vi "QTrkGetSingleResult.vi"(5 "QTrk Instance":T4={"QTrk Pointer"=0, "QTrk Settings"={"Image width"=150, "Image height"=150, "Number of threads (CPU based)"=-1, "Max Queue Size"=128, "XCOR Profile Length"=32, "XCOR Profile Width"=2, "XCOR Iterations"=5, "ZLUT MinRadius"=50.0, "ZLUT MaxRadius"=64.0, "ZLUT AngularSteps"=0, "QI Iterations"=64, "QI RadialSteps"=64, "QI AngularSteps Per Quadrant"=2, "QI MinRadius"=50.0, "QI MaxRadius"=50.0, "CUDA Device# (if using cuda)"=0, "COM Background correction factor"=2.0, "ZLUT RadialSteps"=32, "Gaussian 2D Fit Iterations"=8}}) -> (0 "HasResult":bool, 1 "result":T1, 2 "QTrk Instance":T4={"QTrk Pointer"=0, "QTrk Settings"={"Image width"=150, "Image height"=150, "Number of threads (CPU based)"=-1, "Max Queue Size"=128, "XCOR Profile Length"=32, "XCOR Profile Width"=2, "XCOR Iterations"=5, "ZLUT MinRadius"=50.0, "ZLUT MaxRadius"=64.0, "ZLUT AngularSteps"=0, "QI Iterations"=64, "QI RadialSteps"=64, "QI AngularSteps Per Quadrant"=2, "QI MinRadius"=50.0, "QI MaxRadius"=50.0, "CUDA Device# (if using cuda)"=0, "COM Background correction factor"=2.0, "ZLUT RadialSteps"=32, "Gaussian 2D Fit Iterations"=8}})   [LabVIEW 2011]
uses:
  QTrkInstance.ctl
  QTrkSettings.ctl
  QTrkLocalizationResult.ctl
  QTrkLocalizationJob.ctl
  XYZf.ctl
  QTrkDLL.vi
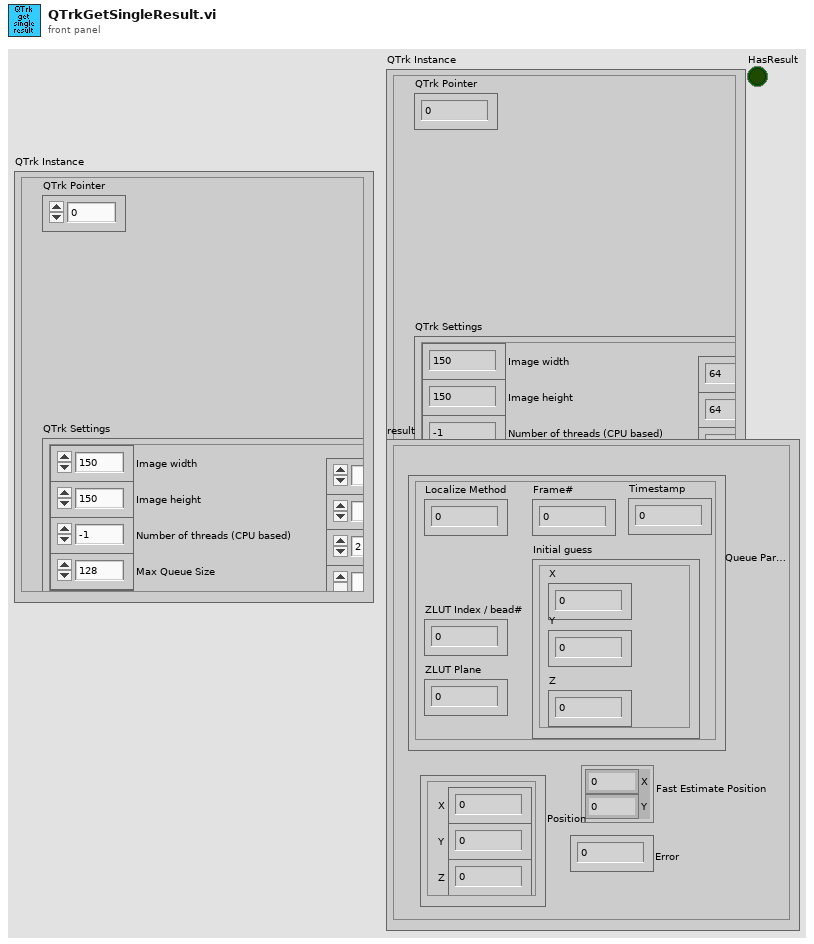
[diagram p1: front panel]
types:
  T1 = typedef "QTrkLocalizationResult.ctl" = cluster{"Queue Params":T2, "Position":T3, "Fast Estimate Position":cluster{"X":sgl, "Y":sgl}, "Error":i32}
  T2 = typedef "QTrkLocalizationJob.ctl" = cluster{"Localize Method":i32, "Frame#":u32, "Timestamp":u32, "ZLUT Index / bead#":i32, "ZLUT Plane":i32, "Initial guess":T3}
  T3 = typedef "XYZf.ctl" = cluster{"X":sgl, "Y":sgl, "Z":sgl}
  T4 = typedef "QTrkInstance.ctl" = cluster{"QTrk Pointer":u64, "QTrk Settings":T5}
  T5 = typedef "QTrkSettings.ctl" = cluster{"Image width":i32, "Image height":i32, "Number of threads (CPU based)":i32, "Max Queue Size":i32, "XCOR Profile Length":i32, "XCOR Profile Width":i32, "XCOR Iterations":i32, "ZLUT MinRadius":sgl, "ZLUT MaxRadius":sgl, "ZLUT AngularSteps":i32, "QI Iterations":i32, "QI RadialSteps":i32, "QI AngularSteps Per Quadrant":i32, "QI MinRadius":sgl, "QI MaxRadius":sgl, "CUDA Device# (if using cuda)":i32, "COM Background correction factor":sgl, "ZLUT RadialSteps":i32, "Gaussian 2D Fit Iterations":i32}
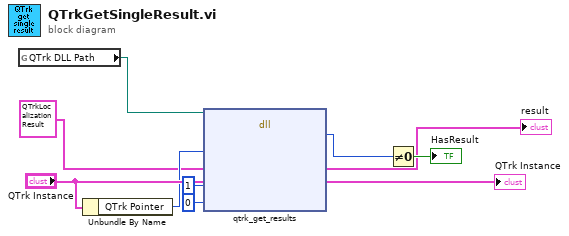
[diagram p0: block diagram]
diagram:
  n1 = global read "QTrkDLL.vi" "QTrk DLL Path"() -> (w9:path)
  n2 = Unbundle By Name("QTrk Instance") -> ("QTrk Pointer"=w7:u64)
  n3 = dll-call lib="D:/jcnossen1/cudaqi-tracker/bin/jtrk-labview.dll" fn="qtrk_get_results"(path in=w9, "tracker"=w7, "results"=T1 {"Queue Params"={"Localize Method"=0, "Frame#"=0, "Timestamp"=0, "ZLUT Index / bead#"=0, "ZLUT Plane"=0, "Initial guess"={"X"=0.0, "Y"=0.0, "Z"=0.0}}, "Position"={"X"=0.0, "Y"=0.0, "Z"=0.0}, "Fast Estimate Position"={"X"=0.0, "Y"=0.0}, "Error"=0} ("Localization Result"), "maxResults"=1, "sortByID"=0) -> ("resultCount"=w3:i32, "results"=→"result":T1)  [unwired: 5 in, 2 out]
  n4 = Not Equal To 0?(x=w3) -> (x != 0?=→"HasResult":bool)
  "QTrk Instance" <- "QTrk Instance"
